vi "test guid wrap and unwrap.vi"() -> ()   [LabVIEW 2013, in "TBM Tests.lvlib"]
uses:
  TBM Tests.lvlib
  root configuration/wrap data.vi
  root configuration/unwrap data.vi
  root configuration/create GUID.vi
  root configuration/TBM configuration.lvclass
panel:
  out "bad":T1(array[cluster])
  out "ok":bool
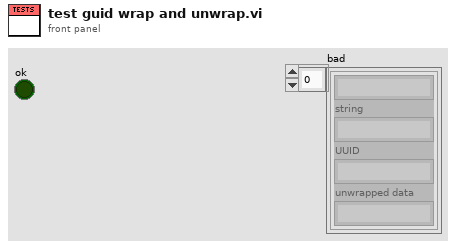
[diagram p1: front panel]
types:
  T1 = cluster{string, "string":string, "UUID":string, "unwrapped data":string}[]
  T2 = cluster{string, "uuid":string, "string":string, "unwrapped data":string}
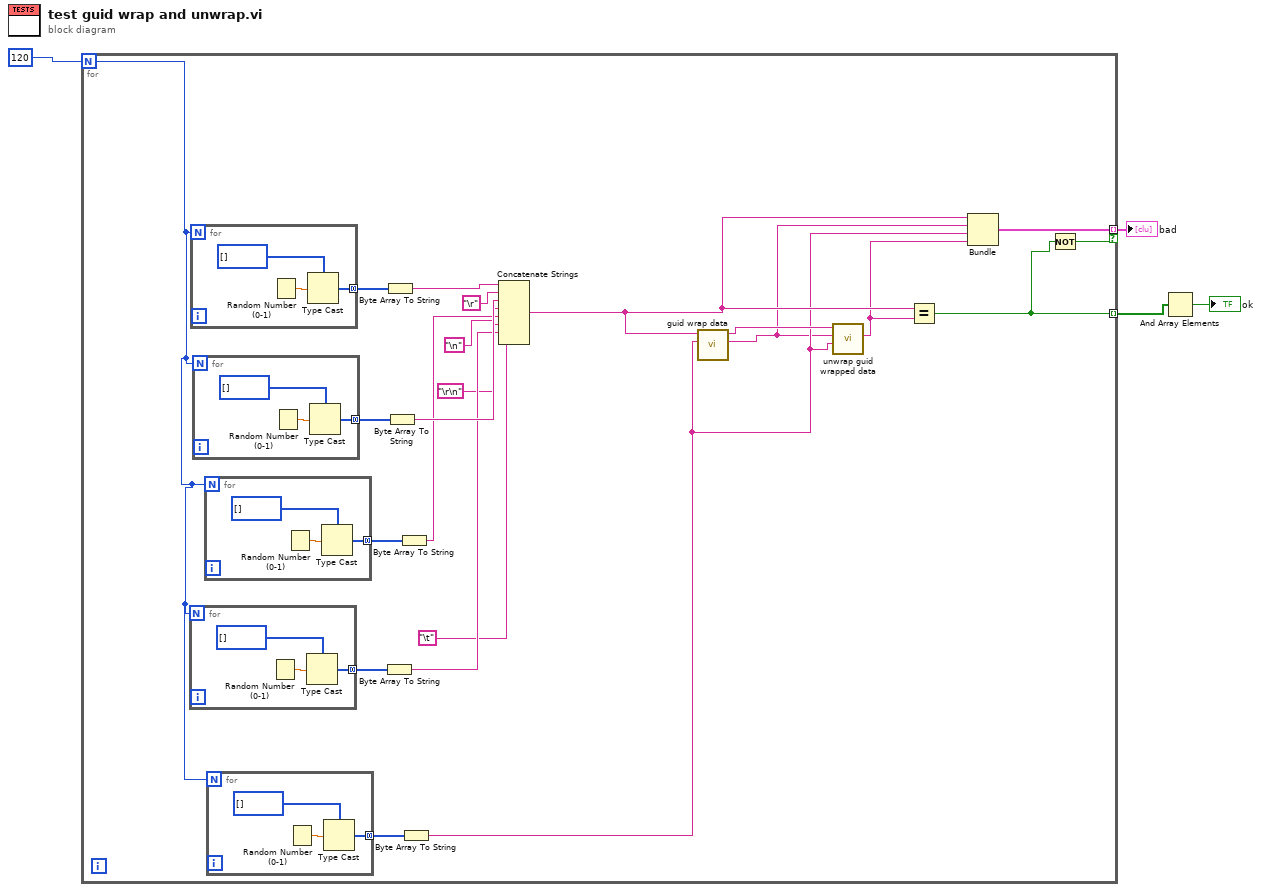
[diagram p0: block diagram]
diagram:
  n1 = for {
    N: 120 -> [w13]
    tunnel: [w10] -> w3 mode=indexing
    tunnel: [w11] -> w1 mode=indexing if=w9
    n2 = for {
      N: w13 -> [_]
      tunnel: [w30] -> w23 mode=concatenating
      n3 = Random Number (0-1)() -> (number: 0 to 1=w32:dbl)
      n4 = Type Cast(type=u8[] [], x=w32) -> (*(type *) &x=w30:u8[])
    }
    n5 = for {
      N: w13 -> [_]
      tunnel: [w39] -> w26 mode=concatenating
      n6 = Random Number (0-1)() -> (number: 0 to 1=w41:dbl)
      n7 = Type Cast(type=u8[] [], x=w41) -> (*(type *) &x=w39:u8[])
    }
    n8 = for {
      N: w13 -> [_]
      tunnel: [w36] -> w25 mode=concatenating
      n9 = Random Number (0-1)() -> (number: 0 to 1=w38:dbl)
      n10 = Type Cast(type=u8[] [], x=w38) -> (*(type *) &x=w36:u8[])
    }
    n11 = for {
      N: w13 -> [_]
      tunnel: [w33] -> w24 mode=concatenating
      n12 = Random Number (0-1)() -> (number: 0 to 1=w35:dbl)
      n13 = Type Cast(type=u8[] [], x=w35) -> (*(type *) &x=w33:u8[])
    }
    n14 = for {
      N: w13 -> [_]
      tunnel: [w27] -> w14 mode=concatenating
      n15 = Random Number (0-1)() -> (number: 0 to 1=w29:dbl)
      n16 = Type Cast(type=u8[] [], x=w29) -> (*(type *) &x=w27:u8[])
    }
    n17 = Byte Array To String(unsigned byte array=w23) -> (string=w19:string)
    n18 = Byte Array To String(unsigned byte array=w26) -> (string=w22:string)
    n19 = Byte Array To String(unsigned byte array=w25) -> (string=w21:string)
    n20 = Byte Array To String(unsigned byte array=w24) -> (string=w20:string)
    n21 = Byte Array To String(unsigned byte array=w14) -> (string=w7:string)
    n22 = Concatenate Strings(w22, "\r", w21, "\n", w20, "\r\n", w19, "\t") -> (w12:string)
    n23 = call "guid wrap data.vi"("identifier"=w7, "data to wrap"=w12) -> ("uuid"=w6:string, "wrapped data"=w8:string)  [unwired: 8 in]
    n24 = call "unwrap guid wrapped data.vi"("identifier"=w7, "uuid"=w6, "data to unwrap"=w8) -> ("unwrapped data"=w5:string)  [unwired: 7 in, 1 out]
    n25 = Equal?(x=w12, y=w5) -> (x = y?=w10:bool)
    n26 = Bundle(w12, "uuid"=w6, "string"=w7, "unwrapped data"=w5) -> (w11:T2)  [unwired: 1 in]
    n27 = Not(x=w10) -> (.not. x?=w9:bool)
  }
  "bad" <- w1
  n28 = And Array Elements(Boolean array=w3) -> (logical AND=→"ok":bool)
